vi "Log Command Drive Path.vi"   [LabVIEW 2016]
uses:
  Global Variables/Drive Path Logging Data.vi
  Global Variables/MotionProfile.vi
  Global Variables/Folder Names.vi
types:
  T1 = typedef "MotionProfile TypeDef.ctl" = cluster{"Left MP Array":dbl[][], "Left MP Index":dbl, "Semaphore":bool, "Right MP Array":dbl[][], "Right MP Index":dbl}
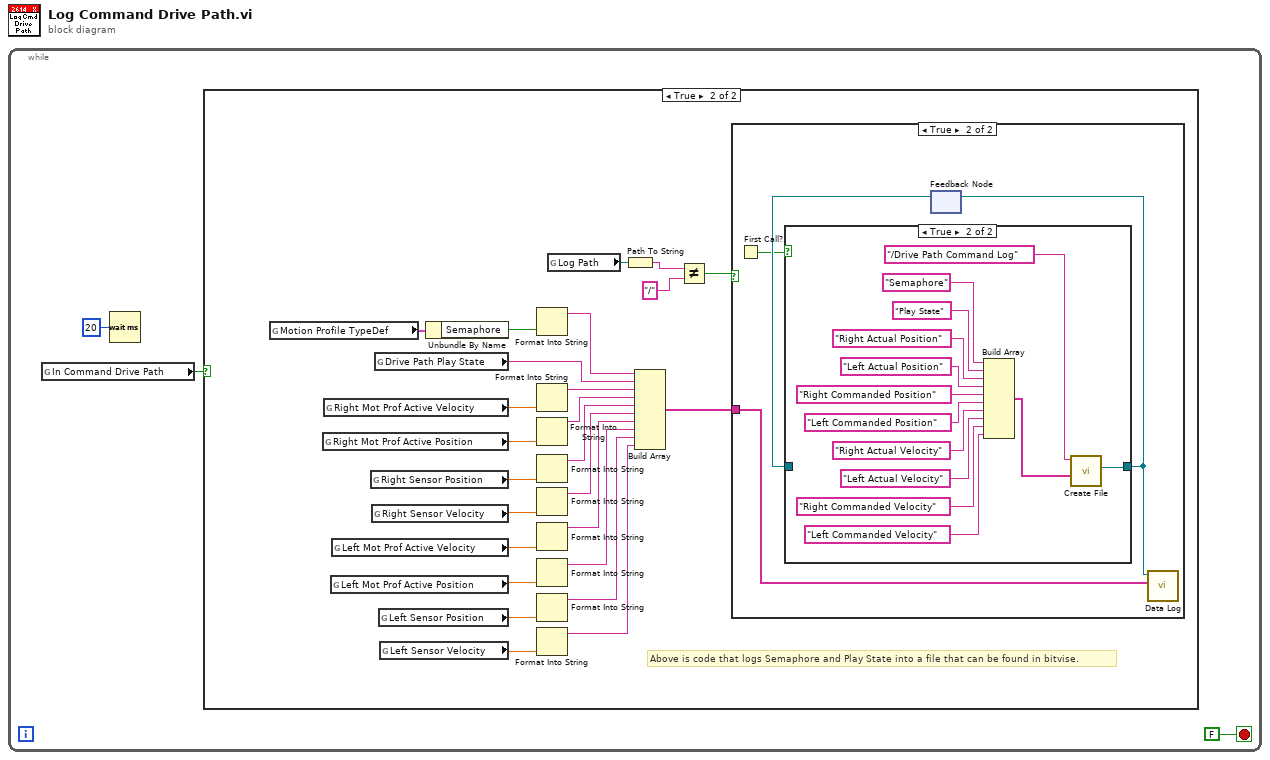
[diagram p0: block diagram]
diagram:
  n1 = while {
    stop <- FALSE stop-if-true
    n2 = global read "Drive Path Logging Data.vi" "In Command Drive Path"() -> (w3:bool)
    n3 = Wait (ms)(milliseconds to wait=u32 20) -> ()  [unwired: 1 out]
    n4 = case shown="True" w3 {
      frame False {
      }
      frame True {
        # "Above is code that logs Semaphore and Play State into a file that can be found in bitvise."
        n5 = global read "MotionProfile.vi" "Motion Profile TypeDef"() -> (w28:T1)
        n6 = global read "Drive Path Logging Data.vi" "Right Mot Prof Active Position"() -> (w10:dbl)
        n7 = global read "Drive Path Logging Data.vi" "Right Mot Prof Active Velocity"() -> (w11:dbl)
        n8 = global read "Drive Path Logging Data.vi" "Left Mot Prof Active Position"() -> (w7:dbl)
        n9 = global read "Drive Path Logging Data.vi" "Left Mot Prof Active Velocity"() -> (w6:dbl)
        n10 = global read "Drive Path Logging Data.vi" "Right Sensor Position"() -> (w4:dbl)
        n11 = global read "Drive Path Logging Data.vi" "Right Sensor Velocity"() -> (w5:dbl)
        n12 = global read "Drive Path Logging Data.vi" "Drive Path Play State"() -> (w12:string)
        n13 = global read "Drive Path Logging Data.vi" "Left Sensor Position"() -> (w8:dbl)
        n14 = global read "Drive Path Logging Data.vi" "Left Sensor Velocity"() -> (w9:dbl)
        n15 = Unbundle By Name(w28) -> ("Semaphore"=w27:bool)
        n16 = Format Into String(w27) -> (resulting string=w26:string)  [unwired: 3 in, 1 out]
        n17 = Format Into String(w11) -> (resulting string=w24:string)  [unwired: 3 in, 1 out]
        n18 = Format Into String(w10) -> (resulting string=w23:string)  [unwired: 3 in, 1 out]
        n19 = Format Into String(w4) -> (resulting string=w22:string)  [unwired: 3 in, 1 out]
        n20 = Format Into String(w5) -> (resulting string=w21:string)  [unwired: 3 in, 1 out]
        n21 = Format Into String(w6) -> (resulting string=w20:string)  [unwired: 3 in, 1 out]
        n22 = Format Into String(w7) -> (resulting string=w19:string)  [unwired: 3 in, 1 out]
        n23 = Format Into String(w8) -> (resulting string=w18:string)  [unwired: 3 in, 1 out]
        n24 = Format Into String(w9) -> (resulting string=w17:string)  [unwired: 3 in, 1 out]
        n25 = global read "Folder Names.vi" "Log Path"() -> (w16:path)
        n26 = Path To String(path=w16) -> (string=w15:string)
        n27 = Build Array(w26, w12, w24, w23, w22, w21, w20, w19, w18, w17) -> (w25:string[])
        n28 = Not Equal?(x=w15, y="/") -> (x != y?=w13:bool)
        n29 = case shown="True" w13 {
          tunnel: w25 -> [_ w29]
          frame False {
          }
          frame True {
            n30 = First Call?() -> (First Call?: T/F=w31:bool)
            n31 = feedback #1() -> (w32:refnum<file>)  [unwired: 1 in]
            n32 = case shown="True" w31 {
              tunnel: [w33 w36] -> w30
              tunnel: w32 -> [w33 _]
              frame False {
              }
              frame True {
                n33 = Build Array("Semaphore" ("File Path/File Name"), "Play State" ("File Path/File Name"), "Right Actual Position" ("File Path/File Name"), "Left Actual Position" ("File Path/File Name"), "Right Commanded Position" ("File Path/File Name"), "Left Commanded Position" ("File Path/File Name"), "Right Actual Velocity" ("File Path/File Name"), "Left Actual Velocity" ("File Path/File Name"), "Right Commanded Velocity" ("File Path/File Name"), "Left Commanded Velocity" ("File Path/File Name")) -> (w34:string[])
                n34 = call "Create File.vi"("Column Titles"=w34, "File Name"="/Drive Path Command Log" ("string")) -> ("File Reference Out"=w36:refnum<file>)  [unwired: 9 in]
              }
            }
            n35 = feedback-in #1(w30) -> ()
            n36 = call "Data Log.vi"("Data In"=w29, "File Reference In"=w30) -> ()  [unwired: 9 in, 1 out]
          }
        }
      }
    }
  }
